vi "set_timings.vi"(8 "error in (no error)":errorcluster, 9 "AOD equilibration time":dbl[unit], 10 "pixel dwell time":dbl[unit], 11 "TrajectoryMG100122AODFrameScan in":refnum<class "TrajectoryMG100122AODFrameScan.lvclass">=refnum) -> (0 "error out":errorcluster, 3 "TrajectoryMG100122AODFrameScan out":refnum<class "TrajectoryMG100122AODFrameScan.lvclass">)   [LabVIEW 2010, in "TrajectoryMG100122AODFrameScan.lvclass"]
uses:
  TrajectoryMG100122AODFrameScan.lvclass
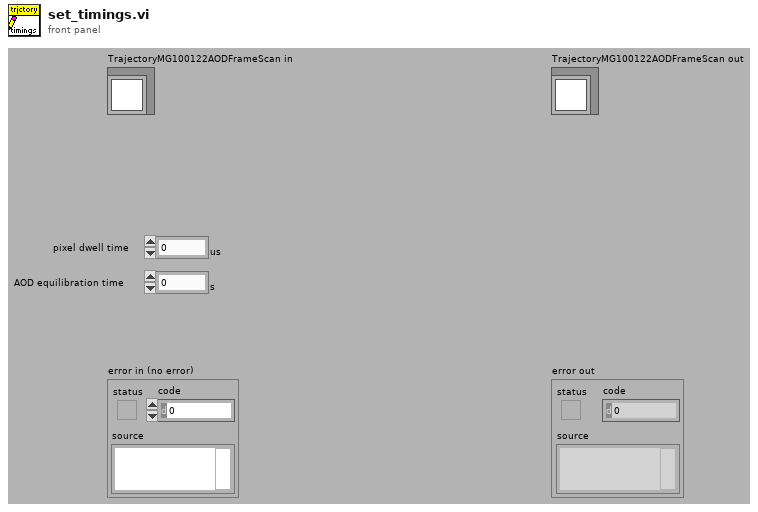
[diagram p1: front panel]
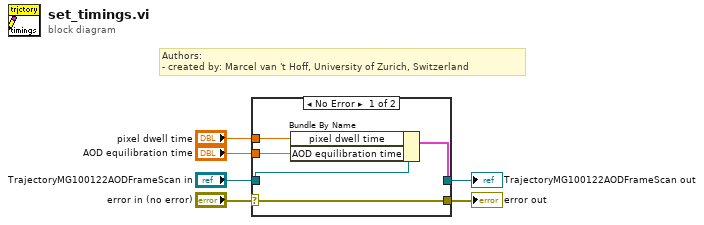
[diagram p0: block diagram]
diagram:
  # "Authors: \n- created by: Marcel van 't Hoff, University of Zurich, Switzerland"
  n1 = case shown="No Error" "error in (no error)" {
    selector: "error in (no error)" -> [w11 w12]
    tunnel: [w11 w12] -> w5
    tunnel: [w9 w13] -> w3
    tunnel: "TrajectoryMG100122AODFrameScan in" -> [w10 w13]
    tunnel: "pixel dwell time" -> [w8 _]
    tunnel: "AOD equilibration time" -> [w7 _]
    frame No Error {
      n2 = Bundle By Name(cluster=w10, "pixel dwell time"=w8, "AOD equilibration time"=w7) -> (w9:cluster{})
    }
    frame Error {
    }
  }
  "error out" <- w5
  "TrajectoryMG100122AODFrameScan out" <- w3
